vi "StripPath.vi"(11 "Path in":path) -> (3 "Path out":path)   [LabVIEW 2012]
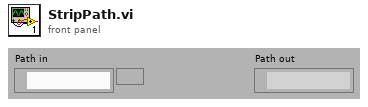
[diagram p1: front panel]
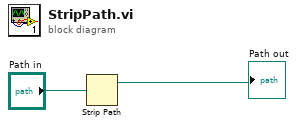
[diagram p0: block diagram]
diagram:
  n1 = Strip Path(path="Path in") -> (stripped path=→"Path out":path)  [unwired: 1 out]
